vi "ProCoDA_external_function.vi"(4 "State":i16, 5 "Time":dbl format="%.2f", 6 "Sensor Values":dbl[](array[numeric]), 7 "Set Points":dbl[](array[numeric])) -> (0 "required data":T1={"Set Point names"=["influent turbidity", "clarified turbidity", "coag_dose", "clarified_target", "", "", "", ""], "required number of setpoints"=4, "required number of sensors"=0, "Sensor names"=[""]}, 3 "output value":dbl)   [LabVIEW 2019]
uses:
  Global Plantita Parameters.vi
panel:
  out "elapsed time":dbl
  out "reset?":bool
  # "Enter the correct information for this control code in the required data structure below. Then make the current value default by right clicking on the border of the data structure. Select \"data operations\" and then select \"make current value default\". These values will be displayed by process controller."
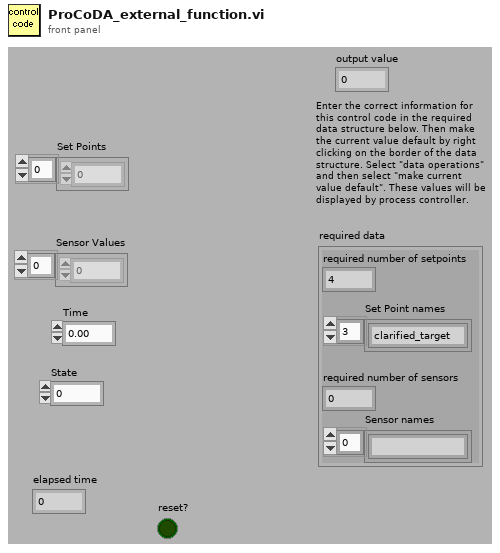
[diagram p1: front panel]
types:
  T1 = cluster{"Set Point names":string[], "required number of setpoints":u8, "required number of sensors":u8, "Sensor names":string[]}
  T2 = cluster{"height_ff (m)":dbl, "C_coag_stock (g/L)":dbl, "flocculation_time(min)":dbl, "clarification_time(min)":dbl, "data_interval (min)":dbl, "kpf":dbl, "kc":dbl, "q":dbl}
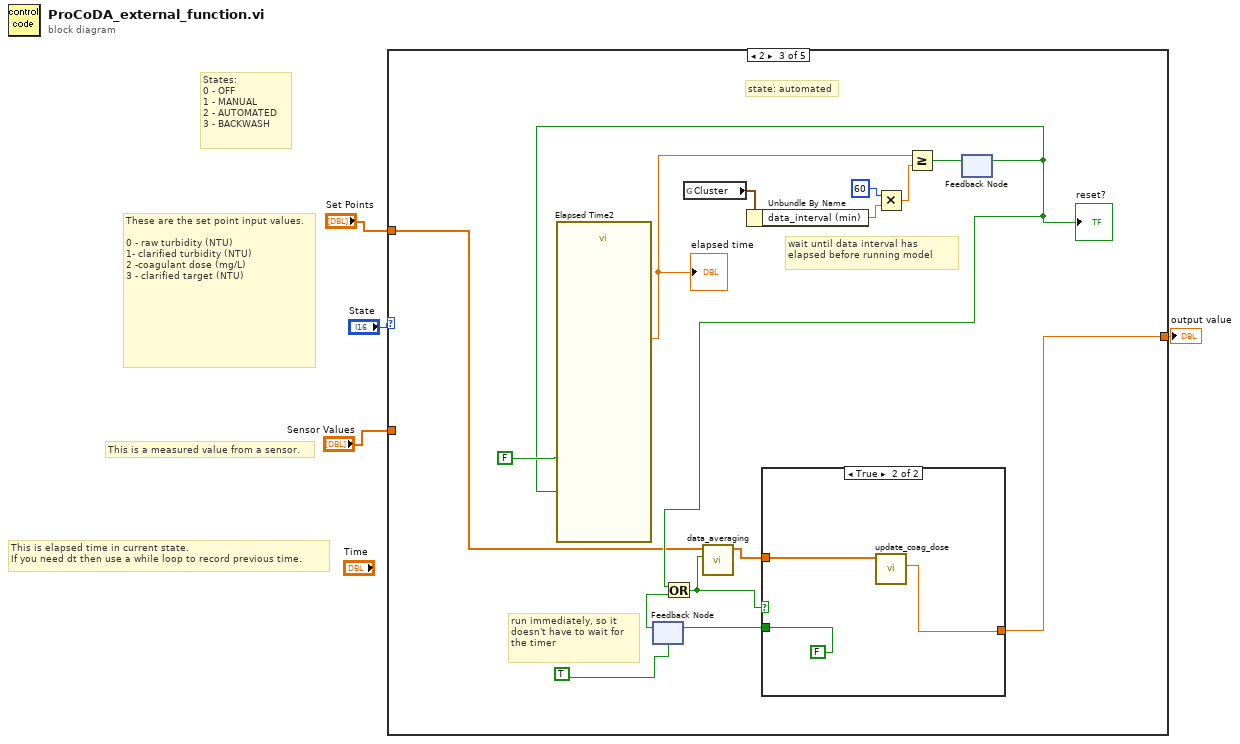
[diagram p0: block diagram]
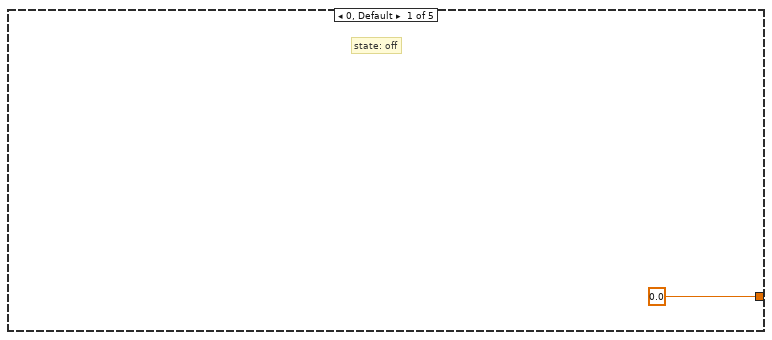
[diagram p2: hidden frame]
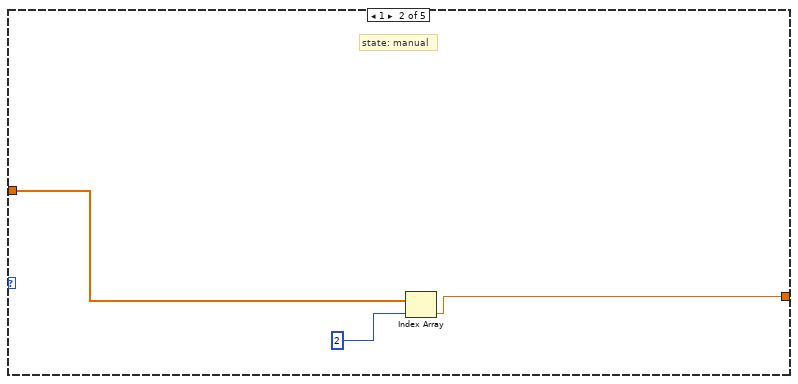
[diagram p3: hidden frame]
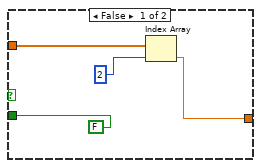
[diagram p4: hidden frame]
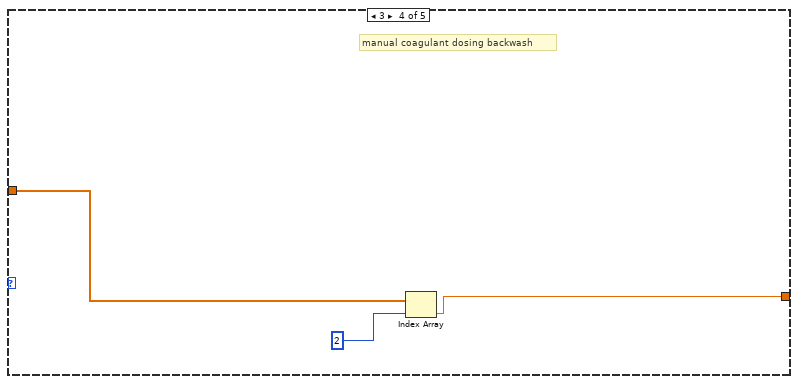
[diagram p5: hidden frame]
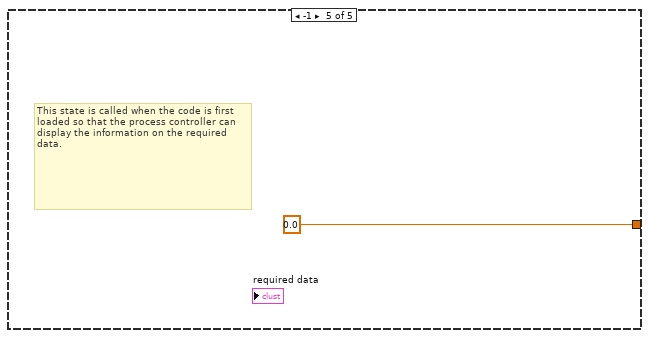
[diagram p6: hidden frame]
diagram:
  # "States:\n0 - OFF\n1 - MANUAL\n2 - AUTOMATED\n3 - BACKWASH"
  # "These are the set point input values.\n\n0 - raw turbidity (NTU)\n1- clarified turbidity (NTU)\n2 -coagulant dose (mg/L)\n3 - clarified target (NTU)"
  # "This is a measured value from a sensor."
  # "This is elapsed time in current state.\nIf you need dt then use a while loop to record previous time."
  n1 = case shown="2" "State" {
    tunnel: "Set Points" -> [_ w7 w11 w32 _]
    tunnel: "Sensor Values" -> [_ _ _ _ _]
    tunnel: [0.0 w6 w21 w31 0.0 ("fraction on")] -> w1
    frame 0, Default {
      # "state: off"
    }
    frame 1 {
      # "state: manual"
      n2 = Index Array(array=w7, index=2) -> (element=w6:dbl)
    }
    frame 2 {
      # "wait until data interval has elapsed before running model"
      # "run immediately, so it doesn't have to wait for the timer"
      # "state: automated"
      n3 = feedback #1(TRUE) -> (w12:bool)
      n4 = global read "Global Plantita Parameters.vi" "Cluster"() -> (w19:T2)
      n5 = Unbundle By Name(w19) -> ("data_interval (min)"=w18:dbl)
      n6 = Multiply(x=60, y=w18) -> (x*y=w16:dbl)
      n7 = feedback #2() -> (w14:bool)  [unwired: 1 in]
      "reset?" <- w14
      n8 = call "Elapsed Time2"("Reset"=w14, "Auto Reset"=FALSE) -> ("Elapsed Time (s)"=w20:dbl)  [unwired: 10 in, 7 out]
      "elapsed time" <- w20
      n9 = Or(x=w14, y=w12) -> (x .or. y?=w9:bool)
      n10 = call "data_averaging.vi"("Reset?"=w9, "New data"=w11) -> ("Output (averaged)"=w10:dbl[])  [unwired: 9 in]
      n11 = case shown="True" w9 {
        tunnel: [w25 w29] -> w21
        tunnel: w10 -> [w27 w30]
        tunnel: [FALSE FALSE] -> w15
        frame False {
          n12 = Index Array(array=w27, index=2) -> (element=w25:dbl)
        }
        frame True {
          n13 = call "update_coag_dose.vi"("Input Array"=w30) -> ("Coagulant_dose [mg/L]"=w29:dbl)  [unwired: 10 in]
        }
      }
      n14 = feedback-in #1(w15) -> ()
      n15 = Greater Or Equal?(x=w20, y=w16) -> (x >= y?=w22:bool)
      n16 = feedback-in #2(w22) -> ()
    }
    frame 3 {
      # "manual coagulant dosing backwash"
      n17 = Index Array(array=w32, index=2) -> (element=w31:dbl)
    }
    frame -1 {
      # "This state is called when the code is first loaded so that the process controller can display the information on the required data."
    }
  }
  "output value" <- w1
